vi "Exercise2.4-FM_RTL-SDR_RX-Problem.vi"() -> ()   [LabVIEW 2013]
uses:
  <vilib>/sound2/lvsound2.llb/Sound Data Format.ctl
  <vilib>/Analysis/2dsp.llb/Rational Resample (single channel, DBL).vi
  <vilib>/sound2/lvsound2.llb/Sound Output Write (DBL Single).vi
  <vilib>/Analysis/NI_AALPro.lvlib
  <instrlib>/rtlsdr/rtlsdr.lvlib
panel:
  out "Spectrum (FFT)":cluster{"f0":dbl, "df":dbl, "magnitude":dbl[]}(graph)
  out "XY Graph":cluster{dbl[], dbl[]}(graph)
  out "DevRefnum":u64
  out "error out":errorcluster
  in  "sound format":T1={"sample rate (S/s)"=44100.0, "number of channels"=1, "bits per sample"=16}
  in  "stop":bool
  in  "Number of Sample":i32=71662
  in  "Center frequency":u32=104300000
  in  "IQ rate":u32=286650
  out "error out":errorcluster
  # "FM Receiver"
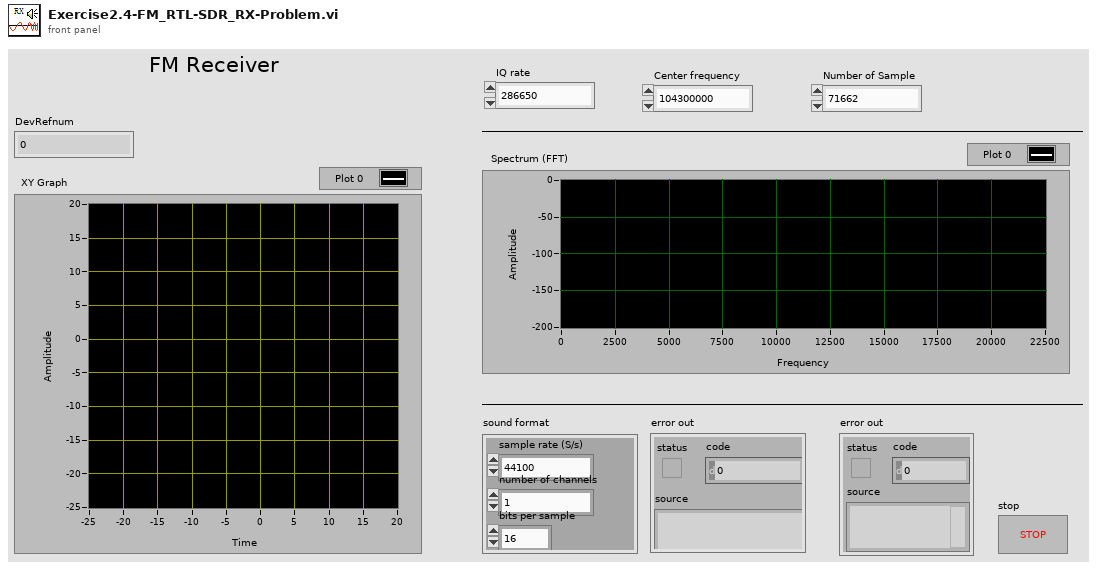
[diagram p1: front panel]
types:
  T1 = typedef "Sound Data Format.ctl" = cluster{"sample rate (S/s)":dbl, "number of channels":i32, "bits per sample":i32}
  T2 = typedef "Sound Output Task ID.ctl" = u32
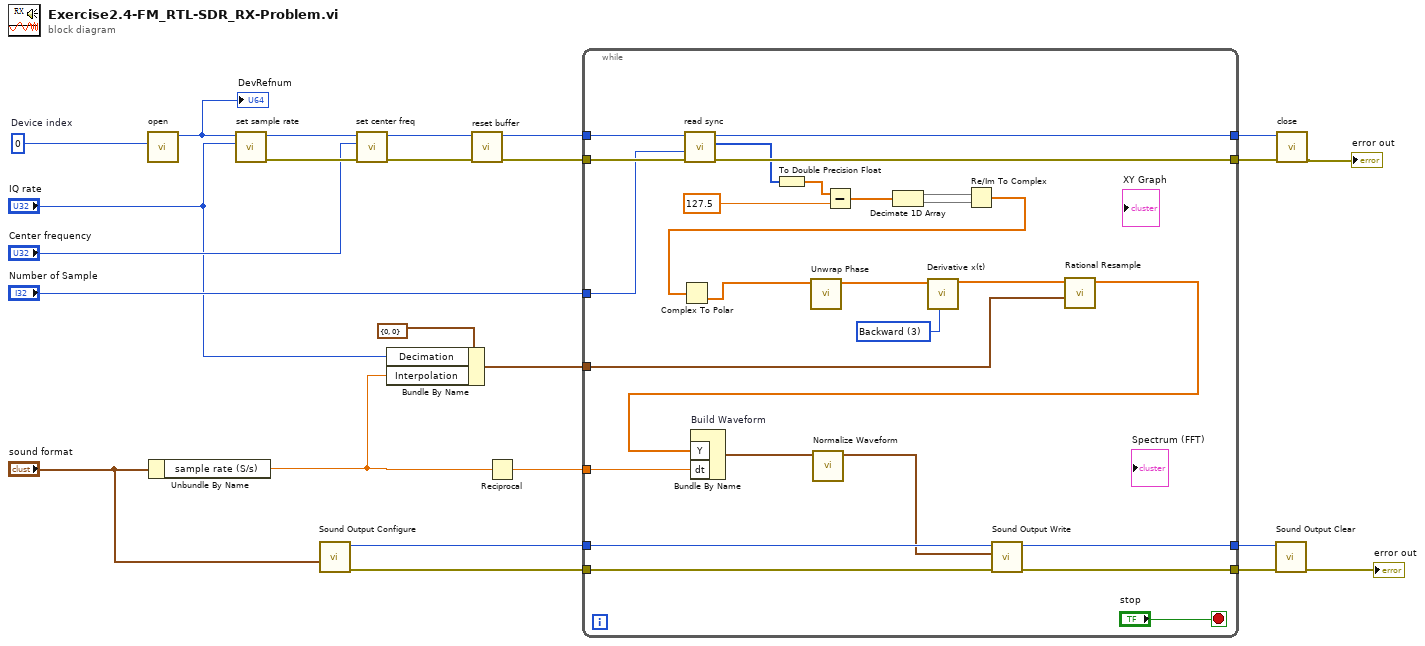
[diagram p0: block diagram]
diagram:
  w17 = u32 0  # Device index
  n1 = call <instrlib>:"open.vi"("index"=w17) -> ("DevRefnum"=w12:u64)  [unwired: 9 in, 1 out]
  "DevRefnum" <- w12
  n2 = Unbundle By Name("sound format") -> ("sample rate (S/s)"=w2:dbl)
  n3 = call <instrlib>:"set sample rate.vi"("rate"="IQ rate", "DevRefnum"=w12) -> ("error out"=w14:errorcluster, "DevRefnum"=w16:u64)  [unwired: 7 in, 1 out]
  n4 = call <vilib>:"Sound Output Configure.vi"("sound format"="sound format") -> ("error out"=w24:errorcluster, "task ID"=w23:T2)  [unwired: 9 in]
  n5 = call <instrlib>:"set center freq.vi"("error in (no error)"=w14, "freq"="Center frequency", "DevRefnum"=w16) -> ("error out"=w13:errorcluster, "DevRefnum"=w15:u64)  [unwired: 6 in, 1 out]
  n6 = Bundle By Name(cluster=cluster{"Interpolation":i32, "Decimation":i32} {"Interpolation"=0, "Decimation"=0}, "Decimation"="IQ rate", "Interpolation"=w2) -> (w1:cluster{"Interpolation":i32, "Decimation":i32})
  n7 = call <instrlib>:"reset buffer.vi"("error in (no error)"=w13, "DevRefnum"=w15) -> ("error out"=w9:errorcluster, "DevRefnum"=w10:u64)  [unwired: 8 in]
  n8 = Reciprocal(x=w2) -> (1/x=w19:dbl)
  n9 = while {
    tunnel: [w39] -> w7
    tunnel: w23 -> [w45]
    tunnel: w24 -> [w44]
    tunnel: [w48] -> w20
    tunnel: [w49] -> w21
    tunnel: w19 -> [w46]
    tunnel: w10 -> [w41]
    tunnel: w9 -> [w40]
    tunnel: [w38] -> w6
    tunnel: "Number of Sample" -> [w35]
    tunnel: w1 -> [w25]
    stop <- "stop" stop-if-true
    w50 = u16 3 items=["2nd Order Central", "4th Order Central", "Forward", "Backward"] ("method")
    n10 = call <instrlib>:"read sync.vi"("error in (no error)"=w40, "len"=w35, "DevRefnum"=w41) -> ("error out"=w38:errorcluster, "buf 2"=w37:u8[], "DevRefnum"=w39:u64)  [unwired: 6 in]
    n11 = To Double Precision Float(number=w37) -> (double precision float=w30:dbl[])
    n12 = Subtract(x=w30, y=127.5) -> (x-y=w32:dbl[])
    n13 = Decimate 1D Array(w32) -> (w34:dbl[], w33:dbl[])
    n14 = Re/Im To Complex(1:w33, 2:w34) -> (0:w36:cdb[])
    n15 = Complex To Polar(r * e^(i*theta)=w36) -> (theta=w42:dbl[])  [unwired: 1 out]
    n16 = call <vilib>:"Unwrap Phase.vi"("Phase"=w42) -> ("Unwrapped Phase"=w43:dbl[])  [unwired: 9 in, 1 out]
    n17 = call <vilib>:"Derivative x(t).vi"("method"=w50, "X"=w43) -> ("dX/dt"=w26:dbl[])  [unwired: 8 in, 1 out]
    n18 = call-poly <vilib>:"Rational Resample.vi"("resample factor"=w25, "X"=w26) -> ("Y"=w27:dbl[])  [unwired: 7 in, 2 out]
    n19 = Bundle By Name "Build Waveform"("Y"=w27, "dt"=w46) -> (w28:waveform(dbl))  [unwired: 1 in]
    n20 = call <vilib>:"Normalize Waveform.vi"("waveform in"=w28) -> ("normalized waveform"=w29:waveform(dbl))  [unwired: 7 in, 3 out]
    n21 = call-poly <vilib>:"Sound Output Write.vi"("error in (no error)"=w44, "data"=w29, "task ID"=w45) -> ("error out"=w48:errorcluster, "task ID out"=w49:T2)  [unwired: 7 in]
  }
  n22 = call <vilib>:"Sound Output Clear.vi"("error in (no error)"=w20, "task ID"=w21) -> ("error out"=→"error out":errorcluster)  [unwired: 9 in]
  n23 = call <instrlib>:"close.vi"("error in (no error)"=w6, "DevRefnum"=w7) -> ("error out"=→"error out":errorcluster)  [unwired: 8 in, 1 out]
